vi "Acquire.vi"(8 "error in (no error)":errorcluster, 9 "Data Queue":refnum<queue>, 10 "Data Notifier":refnum<notifier>, 11 "Hardware Resources in":T1) -> (0 "error out":errorcluster, 3 "Hardware Resources out":T1)   [LabVIEW 2022 SP3, in "pm Acquisition.lvlib"]
doc: "Perform the acquisition. Replace the contents of this diagram with calls to acquisition hardware."
uses:
  pm Acquisition.lvlib
  Hardware Configuration.ctl
  Signal Type.ctl
  <vilib>/express/express signal manip/GetorSetDDTAttributes/Set DDT Attributes/Set DDT Properties.xnode
  <vilib>/express/express shared/transition.llb/Dynamic To Waveform Array.vi
  <vilib>/express/express signal manip/GetorSetDDTAttributes/Set DDT Attributes/SetT0.vi
  <vilib>/express/express shared/transition.llb/Waveform Array To Dynamic.vi
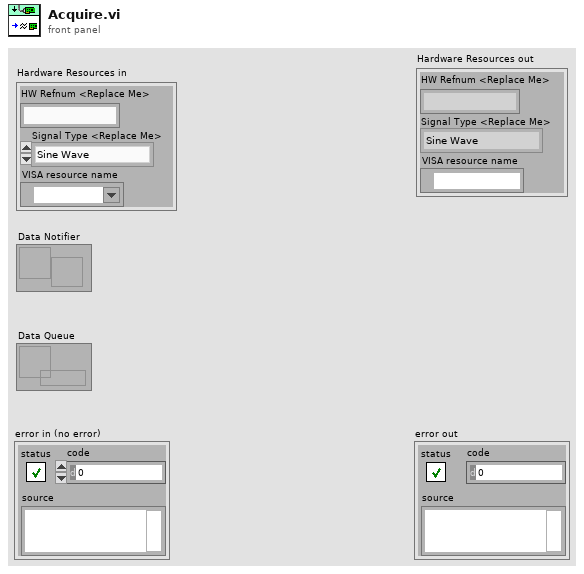
[diagram p1: front panel]
types:
  T1 = typedef "pm Acquisition.lvlib/Hardware Configuration.ctl" = cluster{"HW Refnum <Replace Me>":string, "Signal Type <Replace Me>":T2, "VISA resource name":refnum<visa-resource-name>}
  T2 = typedef "pm Acquisition.lvlib/Signal Type.ctl" = enum16{"Sine Wave", "Square with Noise"}
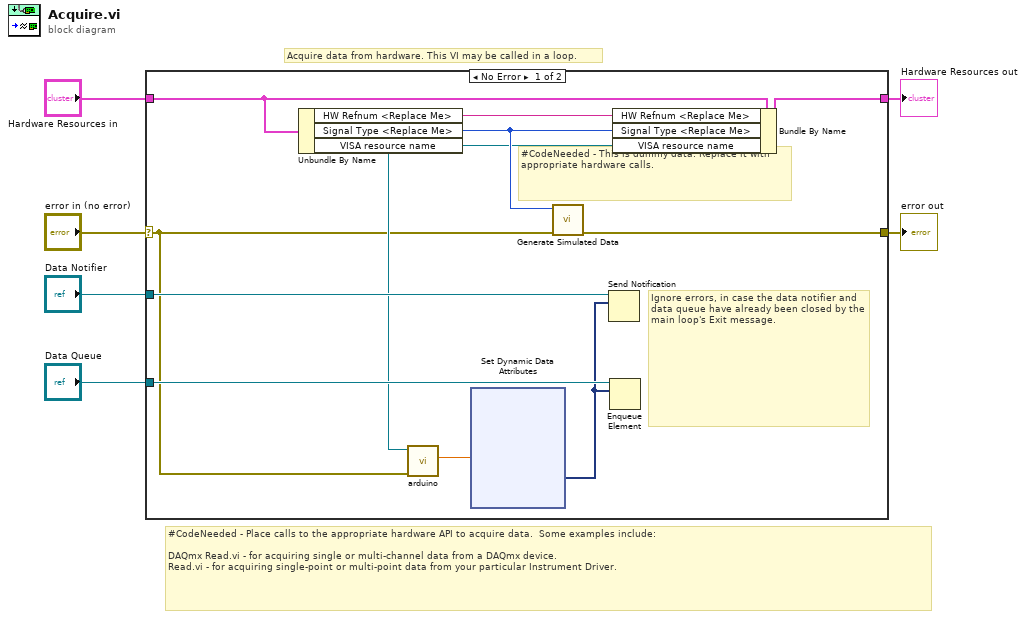
[diagram p0: block diagram]
diagram:
  # "Acquire data from hardware. This VI may be called in a loop."
  # "#CodeNeeded - Place calls to the appropriate hardware API to acquire data.  Some examples include:\n\nDAQmx Read.vi - for acquiring single or multi-channel data from a DAQmx device.\nRead.vi - for acquiring single-point or multi-point data from your particular Instrument Driver."
  n1 = case shown="No Error" "error in (no error)" {
    selector: "error in (no error)" -> [w10 w28]
    tunnel: [w12 w28] -> w5
    tunnel: "Hardware Resources in" -> [w15 w29]
    tunnel: [w17 w29] -> w3
    tunnel: "Data Notifier" -> [w14 _]
    tunnel: "Data Queue" -> [w13 _]
    frame No Error {
      # "Ignore errors, in case the data notifier and data queue have already been closed by the main loop's Exit message."
      # "#CodeNeeded - This is dummy data. Replace it with appropriate hardware calls."
      n2 = Unbundle By Name(w15) -> ("HW Refnum <Replace Me>"=w9:string, "Signal Type <Replace Me>"=w16:T2, "VISA resource name"=w11:refnum<visa-resource-name>)
      n3 = call "arduino.vi"("error in (no error)"=w10, "VISA Refnum in"=w11) -> ("Waveform Chart"=w8:dbl)  [unwired: 8 in, 1 out]
      n4 = xnode "Set Dynamic Data Attributes"("Signals In"=w8) -> ("Signals Out"=w7:dynamicdata)  [unwired: 2 in, 1 out]
      n5 = call "Generate Simulated Data.vi"("error in (no error)"=w10, "Signal Type"=w16) -> ("error out"=w12:errorcluster)  [unwired: 8 in, 1 out]
      n6 = Send Notification(notification=w7, notifier=w14) -> ()  [unwired: 1 in, 2 out]
      n7 = Enqueue Element(queue=w13, element=w7) -> ()  [unwired: 2 in, 3 out]
      n8 = Bundle By Name(cluster=w15, "HW Refnum <Replace Me>"=w9, "Signal Type <Replace Me>"=w16, "VISA resource name"=w11) -> (w17:T1)
    }
    frame Error {
    }
  }
  "Hardware Resources out" <- w3
  "error out" <- w5
